vi "Query Sequencer List All Transition Times.vi"(8 "error in (no error)":errorcluster, 10 "Instance (1)":i32=1, 11 "VISA resource name":refnum<visa-resource-name>) -> (0 "error out":errorcluster, 2 "Transition Times":dbl[](array[numeric]) format="%^.3e", 3 "VISA resource name out":refnum<visa-resource-name>)   [LabVIEW 2015, in "Rohde&Schwarz CMXP GPRF.lvlib"]
doc: "Queries the transition times for all sequencer list entries.\n\nAttribute:\nRSCMXPGPRF_ATTR_SEQUENCER_LIST_ALL_TRANSITION_TIMES\n\nRemote-control command:\nSOURce:GPRF:GEN<i>:SEQuencer:LIST:TTIMe:ALL?"
uses:
  <instrlib>/Rohde&Schwarz CMXP GPRF/Rohde&Schwarz CMXP GPRF.lvlib
  <instrlib>/Rohde&Schwarz CMXP GPRF/Private/rsidr_core.llb/rsidr_core.lvlib
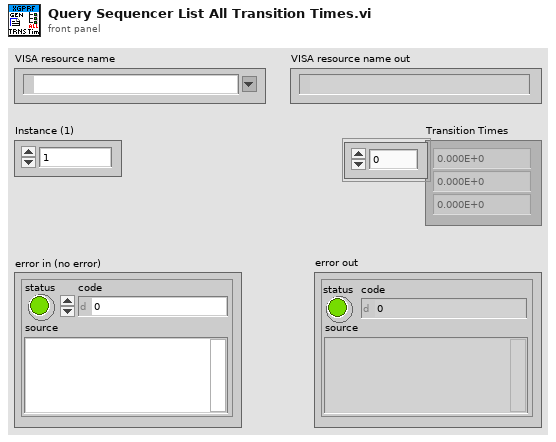
[diagram p1: front panel]
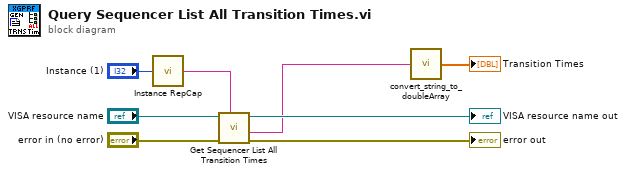
[diagram p0: block diagram]
diagram:
  n1 = call <instrlib>:"Instance RepCap.vi"("instance  in"="Instance (1)") -> ("instance out"=w7:string)
  n2 = call "Get Sequencer List All Transition Times"("Repeated Capabilities"=w7, "error in (no error)"="error in (no error)", "instrument handle"="VISA resource name") -> ("error out"=→"error out":errorcluster, "Sequencer List All Transition Times"=w1:string, "instrument handle out"=→"VISA resource name out":refnum<visa-resource-name>)  [unwired: 6 in]
  n3 = call <instrlib>:"convert_string_to_doubleArray.vi"("string in"=w1) -> ("double array out"=→"Transition Times":dbl[])  [unwired: 3 in, 1 out]
